vi "Teleop.vi"(10 "Match Info":T1={"Autonomous Elapsed Seconds"=0.0, "TeleOp Elapsed Seconds"=0.0, "Disabled Elapsed Seconds"=0.0, "Visited Autonomous"=FALSE, "Visited TeleOp"=FALSE, "Visited Disabled"=FALSE, "Autonomous Settings"={"Autonomous Style"=enum."Independent", "VI Refnum"=refnum}}, 11 "Call Context":T2) -> ()   [LabVIEW 2015]
doc: "This VI is called for each TeleOp packet received from the DS where the robot is not disabled. It is often used to read from the joysticks and update I/O or to update setpoints for timed control loops. It should complete and return within 20 milliseconds or it may miss DS packets."
uses:
  <vilib>/Rock Robotics/WPI/DriverStation/WPI_DriverStationDerivedRobotMode.ctl
  <vilib>/Rock Robotics/WPI/DriverStation/WPI_DriverStationMatch Info.ctl
  <vilib>/Rock Robotics/Network Tables/NT Read Boolean.vi
  <vilib>/Rock Robotics/Network Tables/NT Read Number.vi
  <vilib>/Rock Robotics/WPI/Utilities/WPI_GetSetVariantRefNum.vi
  Robot Global Data.vi
  <vilib>/Rock Robotics/Network Tables/SD Write Boolean.vi
  <vilib>/Rock Robotics/Network Tables/SD Write Number.vi
panel:
  in  "Speed":dbl
  out "Sample Slider 0":dbl(slide) scale=0.0..5.0
  out "Sample Boolean 1":bool
  out "Sample Boolean 0":bool
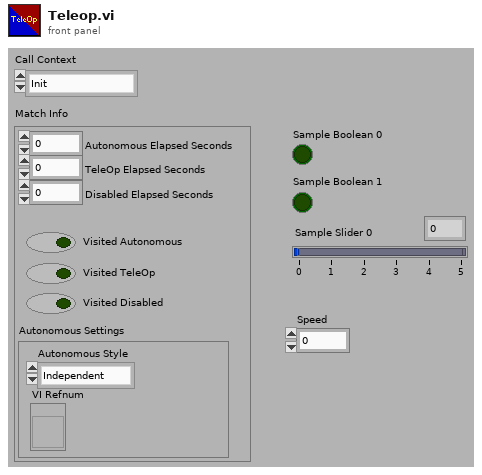
[diagram p1: front panel]
types:
  T1 = typedef "WPI_DriverStationMatch Info.ctl" = cluster{"Autonomous Elapsed Seconds":dbl, "TeleOp Elapsed Seconds":dbl, "Disabled Elapsed Seconds":dbl, "Visited Autonomous":bool, "Visited TeleOp":bool, "Visited Disabled":bool, "Autonomous Settings":cluster{"Autonomous Style":enum16{"Iterative", "Independent"}, "VI Refnum":refnum<vi>}}
  T2 = typedef "WPI_DriverStationDerivedRobotMode.ctl" = enum16{"Init", "Execute", "Stop"}
  T3 = typedef "WPI_JoystickDevRef.ctl" = cluster{"Device":T4}
  T4 = typedef "WPI_JoystickDeviceEnum.ctl" = enum16{"USB 0", "USB 1", "USB 2", "USB 3", "USB 4", "USB 5"}
  T5 = cluster{"Axes[0]":dbl, "Axes[1]":dbl, "Axes[2]":dbl, "Axes[3]":dbl, "Axes[4]":dbl, "Axes[5]":dbl, "Axes[6]":dbl, "Axes[7]":dbl, "Axes[8]":dbl}
  T6 = cluster{"Buttons[0]":bool, "Buttons[1]":bool, "Buttons[2]":bool, "Buttons[3]":bool, "Buttons[4]":bool, "Buttons[5]":bool, "Buttons[6]":bool, "Buttons[7]":bool, "Buttons[8]":bool}
  T7 = typedef "WPI_EncoderDevRef.ctl" = cluster{"DevStatus":errorcluster, "EncoderIndex":T8, "CounterIndex":T9, "DistancePerCount":dbl, "Decoding Type":T10}
  T8 = typedef "FPGA_EncoderIdx.ctl" = enum8{"Enc 0", "Enc 1", "Enc 2", "Enc 3", "Enc 4", "Enc 5", "Enc 6", "Enc 7", "Invalid"}
  T9 = typedef "FPGA_CounterCtrSystemIndex.ctl" = enum8{"Ctr 0", "Ctr 1", "Ctr 2", "Ctr 3", "Ctr 4", "Ctr 5", "Ctr 6", "Ctr 7", "Invalid"}
  T10 = typedef "WPI_EncoderType.ctl" = enum16{"1x", "2x", "4x"}
  T11 = typedef "WPI_RobotDriveDevRef.ctl" = cluster{"DevStatus":errorcluster, "Motors[]":T12[], "Square Inputs":bool, "Max Output":dbl}
  T12 = typedef "WPI_MotorControlDeviceRef.ctl" = cluster{"DeviceStatus":errorcluster, "Type":T13, "PWM":cluster{"PWM Channel":T14, "DeadBand":T15}, "CAN":cluster{"Device Number":u8, "Control Mode":T16, "Semaphore":T17, "Max Vout":dbl, "TalonSRX Control Mode":T18}, "Invert":bool}
  T13 = typedef "WPI_MotorControlType.ctl" = enum16{"PWM", "CAN", "CANTalonSRX"}
  T14 = typedef "FPGA_DIOPWMChannel.ctl" = enum8{"PWM 0", "PWM 1", "PWM 2", "PWM 3", "PWM 4", "PWM 5", "PWM 6", "PWM 7", "PWM 8", "PWM 9", "PWM MXP 0", "PWM MXP 1", "PWM MXP 2", "PWM MXP 3", "PWM MXP 4", "PWM MXP 5", "PWM MXP 6", "PWM MXP 7", "PWM MXP 8", "PWM MXP 9", "Invalid"}
  T15 = typedef "WPI_PWMDeadband.ctl" = cluster{"Name":string, "maxPositivePwm":i32, "minPositivePwm":i32, "centerPwm":i32, "maxNegativePwm":i32, "minNegativePwm":i32, "angularRange":u16}
  T16 = typedef "WPI_CANJaguar_ControlMode.ctl" = enum8{"Percent VBus", "Current", "Speed", "Position", "Voltage"}
  T17 = typedef "Semaphore RefNum" = refnum<k1>
  T18 = typedef "WPI_CANTalonSRX_APIControlMode.ctl" = enum8{"Percent VBus", "Speed", "Position", "Slave", "Unchanged / Invalid", "Voltage Compensation", "Current", "Motion Profile"}
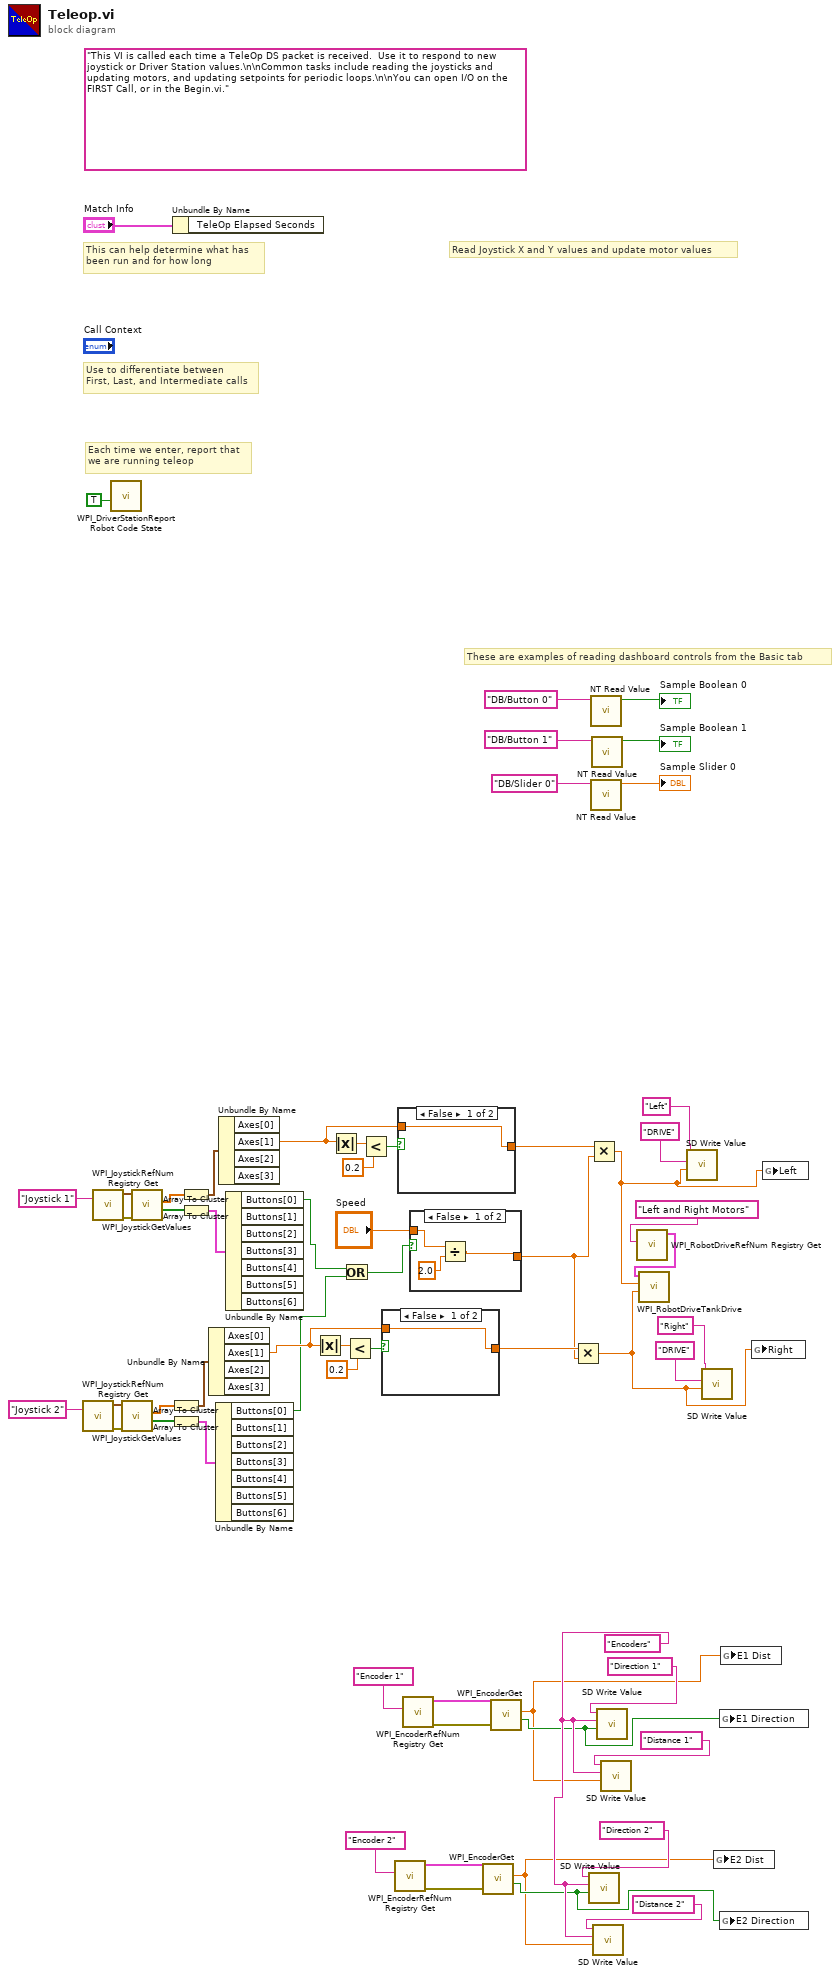
[diagram p0: block diagram]
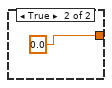
[diagram p3: hidden frame]
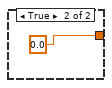
[diagram p4: hidden frame]
diagram:
  w9 = "Encoders"
  (unwired) "This VI is called each time a TeleOp DS packet is received.  Use it to respond to new joystick or Driver Station values.\n\nCommon tasks include reading the joysticks and updating motors, and updating setpoints for periodic loops.\n\nYou can open I/O on the FIRST Call, or in the Begin.vi."
  # "These are examples of reading dashboard controls from the Basic tab"
  # "Each time we enter, report that\nwe are running teleop"
  # "Use to differentiate between\nFirst, Last, and Intermediate calls"
  # "This can help determine what has\nbeen run and for how long"
  # "Read Joystick X and Y values and update motor values"
  n1 = call <vilib>:"WPI_JoystickRefNum Registry Get.vi"("refnum name"="Joystick 2") -> ("error out"=w44:errorcluster, "JoystickDevRef"=w1:T3)  [unwired: 9 in]
  n2 = call <vilib>:"WPI_JoystickRefNum Registry Get.vi"("refnum name"="Joystick 1") -> ("error out"=w51:errorcluster, "JoystickDevRef"=w50:T3)  [unwired: 9 in]
  n3 = call <vilib>:"WPI_DriverStationReport Robot Code State.vi"("TeleOp"=TRUE ("Autonomous")) -> ()  [unwired: 10 in, 1 out]
  n4 = call <vilib>:"WPI_JoystickGetValues.vi"("error in (no error)"=w44, "JoystickDevRef"=w1) -> ("Buttons"=w42:bool[], "Axes"=w43:dbl[])  [unwired: 5 in, 3 out]
  n5 = call <vilib>:"WPI_JoystickGetValues.vi"("error in (no error)"=w51, "JoystickDevRef"=w50) -> ("Buttons"=w48:bool[], "Axes"=w49:dbl[])  [unwired: 5 in, 3 out]
  n6 = Array To Cluster(array=w43) -> (cluster=w41:T5)
  n7 = Array To Cluster(array=w42) -> (cluster=w40:T6)
  n8 = Unbundle By Name("Match Info") -> ()  [unwired: 1 out]
  n9 = Array To Cluster(array=w49) -> (cluster=w47:T5)
  n10 = Array To Cluster(array=w48) -> (cluster=w46:T6)
  n11 = Unbundle By Name(w41) -> ("Axes[1]"=w30:dbl)  [unwired: 3 out]
  n12 = Unbundle By Name(w40) -> ("Buttons[0]"=w21:bool)  [unwired: 6 out]
  n13 = Unbundle By Name(w47) -> ("Axes[1]"=w35:dbl)  [unwired: 3 out]
  n14 = Unbundle By Name(w46) -> ("Buttons[0]"=w22:bool)  [unwired: 6 out]
  n15 = Absolute Value(x=w30) -> (abs(x)=w34:dbl)
  n16 = Absolute Value(x=w35) -> (abs(x)=w39:dbl)
  n17 = Or(x=w22, y=w21) -> (x .or. y?=w20:bool)
  n18 = Less?(x=w34, y=0.2) -> (x < y?=w32:bool)
  n19 = Less?(x=w39, y=0.2) -> (x < y?=w37:bool)
  n20 = case shown="False" w32 {
    tunnel: [w61 0.0] -> w31
    tunnel: w30 -> [w61 _]
    frame False {
    }
    frame True {
    }
  }
  n21 = call <vilib>:"WPI_EncoderRefNum Registry Get.vi"("refnum name"="Encoder 2") -> ("error out"=w13:errorcluster, "EncoderDevRef"=w12:T7)  [unwired: 9 in]
  n22 = case shown="False" w37 {
    tunnel: [w63 0.0] -> w36
    tunnel: w35 -> [w63 _]
    frame False {
    }
    frame True {
    }
  }
  n23 = call <vilib>:"WPI_EncoderRefNum Registry Get.vi"("refnum name"="Encoder 1") -> ("error out"=w18:errorcluster, "EncoderDevRef"=w17:T7)  [unwired: 9 in]
  n24 = case shown="False" w20 {
    tunnel: [w66 w68] -> w29
    tunnel: "Speed" -> [w67 w68]
    frame False {
      n25 = Divide(x=w67, y=2.0) -> (x/y=w66:dbl)
    }
    frame True {
    }
  }
  n26 = call <vilib>:"WPI_EncoderGet.vi"("error in (no error)"=w13, "EncoderDevRef"=w12) -> ("Direction"=w7:bool, "Distance"=w5:dbl)  [unwired: 4 in, 4 out]
  n27 = call <vilib>:"WPI_EncoderGet.vi"("error in (no error)"=w18, "EncoderDevRef"=w17) -> ("Direction"=w8:bool, "Distance"=w6:dbl)  [unwired: 4 in, 4 out]
  n28 = Multiply(x=w31, y=w29) -> (x*y=w2:dbl)
  n29 = Multiply(x=w36, y=w29) -> (x*y=w3:dbl)
  n30 = call-poly <vilib>:"SD Write Value.vi"("Boolean"=w7, "Table Prefix"=w9, "Name"="Direction 2") -> ()  [unwired: 7 in, 2 out]
  n31 = call-poly <vilib>:"NT Read Value.vi"("Name"="DB/Button 0" ("refnum name")) -> ("Boolean"=→"Sample Boolean 0":bool)  [unwired: 9 in, 1 out]
  n32 = call-poly <vilib>:"NT Read Value.vi"("Name"="DB/Slider 0" ("refnum name")) -> ("Numeric"=→"Sample Slider 0":dbl)  [unwired: 9 in, 1 out]
  n33 = call-poly <vilib>:"NT Read Value.vi"("Name"="DB/Button 1" ("refnum name")) -> ("Boolean"=→"Sample Boolean 1":bool)  [unwired: 9 in, 1 out]
  n34 = call-poly <vilib>:"SD Write Value.vi"("Numeric"=w5, "Table Prefix"=w9, "Name"="Distance 2") -> ()  [unwired: 7 in, 2 out]
  n35 = call-poly <vilib>:"SD Write Value.vi"("Boolean"=w8, "Table Prefix"=w9, "Name"="Direction 1") -> ()  [unwired: 7 in, 2 out]
  n36 = call-poly <vilib>:"SD Write Value.vi"("Numeric"=w6, "Table Prefix"=w9, "Name"="Distance 1") -> ()  [unwired: 7 in, 2 out]
  n37 = call <vilib>:"WPI_RobotDriveRefNum Registry Get.vi"("refnum name"="Left and Right Motors") -> ("RobotDriveDevRef"=w28:T11)  [unwired: 9 in, 1 out]
  n38 = call <vilib>:"WPI_RobotDriveTankDrive.vi"("Right axis value"=w2, "Left axis value"=w3, "RobotDriveDevRef"=w28) -> ()  [unwired: 6 in, 3 out]
  n39 = call-poly <vilib>:"SD Write Value.vi"("Numeric"=w3, "Table Prefix"="DRIVE", "Name"="Left") -> ()  [unwired: 7 in, 2 out]
  n40 = call-poly <vilib>:"SD Write Value.vi"("Numeric"=w2, "Table Prefix"="DRIVE", "Name"="Right") -> ()  [unwired: 7 in, 2 out]
  n41 = global write "Robot Global Data.vi" "E2 Dist"(w5) -> ()
  n42 = global write "Robot Global Data.vi" "E1 Direction"(w8) -> ()
  n43 = global write "Robot Global Data.vi" "E2 Direction"(w7) -> ()
  n44 = global write "Robot Global Data.vi" "E1 Dist"(w6) -> ()
  n45 = global write "Robot Global Data.vi" "Right"(w2) -> ()
  n46 = global write "Robot Global Data.vi" "Left"(w3) -> ()
